vi "Set Conrtrol ID.vi"(8 "error in (no error)":errorcluster, 11 "GUI Control in":refnum<class "GUI Control.lvclass">) -> (0 "error out":errorcluster, 3 "GUI Control out":refnum<class "GUI Control.lvclass">)   [LabVIEW 2015, in "GUI Control.lvclass"]
uses:
  GUI Control.lvclass
  GUI Control.lvclass/GUI Control.ctl
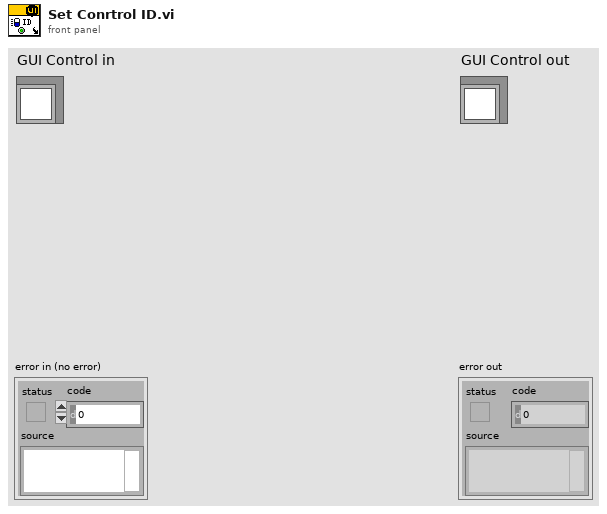
[diagram p1: front panel]
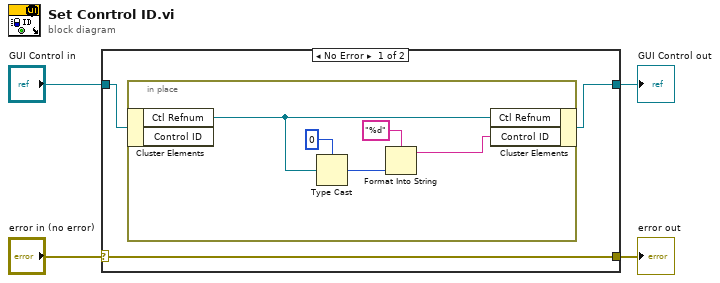
[diagram p0: block diagram]
diagram:
  n1 = case shown="No Error" "error in (no error)" {
    selector: "error in (no error)" -> [w7 w13]
    tunnel: [w7 w13] -> w3
    tunnel: [w5 w14] -> w1
    tunnel: "GUI Control in" -> [w6 w14]
    frame No Error {
      n2 = in-place {
        n3 = in-place-cluster #1(w6) -> ("Ctl Refnum"=w11:refnum<vi>)  [unwired: 1 out]
        n4 = Type Cast(type=u16 0, x=w11) -> (*(type *) &x=w9:u16)
        n5 = Format Into String(format string="%d", w9) -> (resulting string=w8:string)  [unwired: 2 in, 1 out]
        n6 = in-place-cluster #1("Ctl Refnum"=w11, "Control ID"=w8) -> (w5:refnum<class "GUI Control.lvclass">)
      }
    }
    frame Error {
    }
  }
  "error out" <- w3
  "GUI Control out" <- w1
